vi "wait Targets match.vi"(10 "status":T2, 11 "Mercury Targets":T1) -> (1 "Target AND Rate Match":bool, 2 "Target ~ Magnet":bool, 3 "Target ~ PS":bool)   [LabVIEW 2016, in "Instrument.OxfordVRM.lvclass"]
uses:
  Instrument.OxfordVRM.lvclass
  Typedefs/Status.ctl
  Typedefs/Targets.ctl
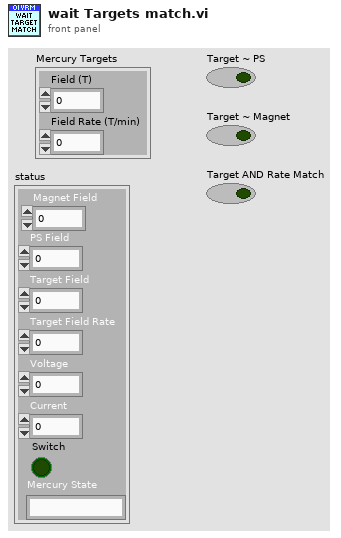
[diagram p1: front panel]
types:
  T1 = typedef "Instrument.OxfordVRM.lvclass/Targets.ctl" = cluster{"Field (T)":dbl, "Field Rate (T/min)":dbl}
  T2 = typedef "Instrument.OxfordVRM.lvclass/Status.ctl" = cluster{"Magnet Field":dbl, "PS Field":dbl, "Target Field":dbl, "Target Field Rate":dbl, "Voltage":dbl, "Current":dbl, "Switch":bool, "Mercury State":string}
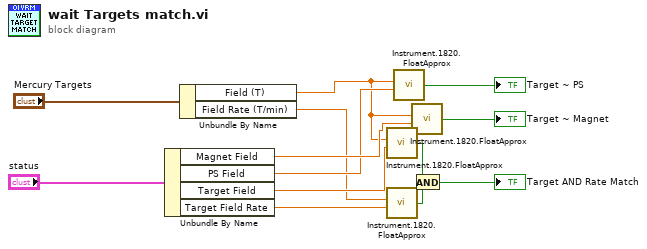
[diagram p0: block diagram]
diagram:
  n1 = Unbundle By Name("status") -> ("Magnet Field"=w12:dbl, "PS Field"=w11:dbl, "Target Field"=w10:dbl, "Target Field Rate"=w7:dbl)
  n2 = Unbundle By Name("Mercury Targets") -> ("Field (T)"=w2:dbl, "Field Rate (T/min)"=w9:dbl)
  n3 = call "Instrument.1820.FloatApprox.vi"("y"=w10, "x"=w2) -> ("x ~ y?"=w6:bool)  [unwired: 4 in]
  n4 = call "Instrument.1820.FloatApprox.vi"("y"=w7, "x"=w9) -> ("x ~ y?"=w8:bool)  [unwired: 4 in]
  n5 = call "Instrument.1820.FloatApprox.vi"("y"=w11, "x"=w2) -> ("x ~ y?"=→"Target ~ PS":bool)  [unwired: 4 in]
  n6 = call "Instrument.1820.FloatApprox.vi"("y"=w12, "x"=w2) -> ("x ~ y?"=→"Target ~ Magnet":bool)  [unwired: 4 in]
  n7 = And(x=w6, y=w8) -> (x .and. y?=→"Target AND Rate Match":bool)
